vi "Check Test Report.vi"(8 "error in (no error)":errorcluster) -> (0 "error out":errorcluster)   [LabVIEW 2021]
uses:
  <vilib>/addons/_JKI Toolkits/Caraya/classes/Properties.Test/Properties.Test.lvclass
  C:/Program Files (x86)/National Instruments/LabVIEW 2021/vi.lib/addons/_JKI Toolkits/Caraya/classes/Properties/Properties.lvclass
  <vilib>/addons/_JKI Toolkits/Caraya/classes/Properties.Assert/Properties.Assert.lvclass
  <vilib>/Utility/file.llb/Read Delimited Spreadsheet (string).vi
  <vilib>/addons/_JKI Toolkits/Caraya/classes/Assert/Assert Equal Value_Variant.vi
  <vilib>/addons/_JKI Toolkits/Caraya/classes/Assert/Assert Greater Or Equal_Variant.vi
  <vilib>/addons/_JKI Toolkits/Caraya/classes/Assert/Assert True.vi
  <vilib>/addons/_JKI Toolkits/Caraya/classes/Test/Test.lvclass
  <vilib>/addons/_JKI Toolkits/Caraya/classes/Assert/Assert.lvclass
  <vilib>/addons/_JKI Toolkits/Caraya/classes/Properties/Properties.lvclass
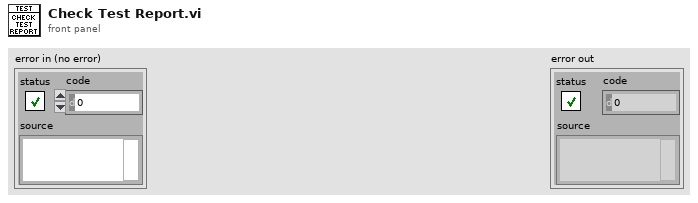
[diagram p1: front panel]
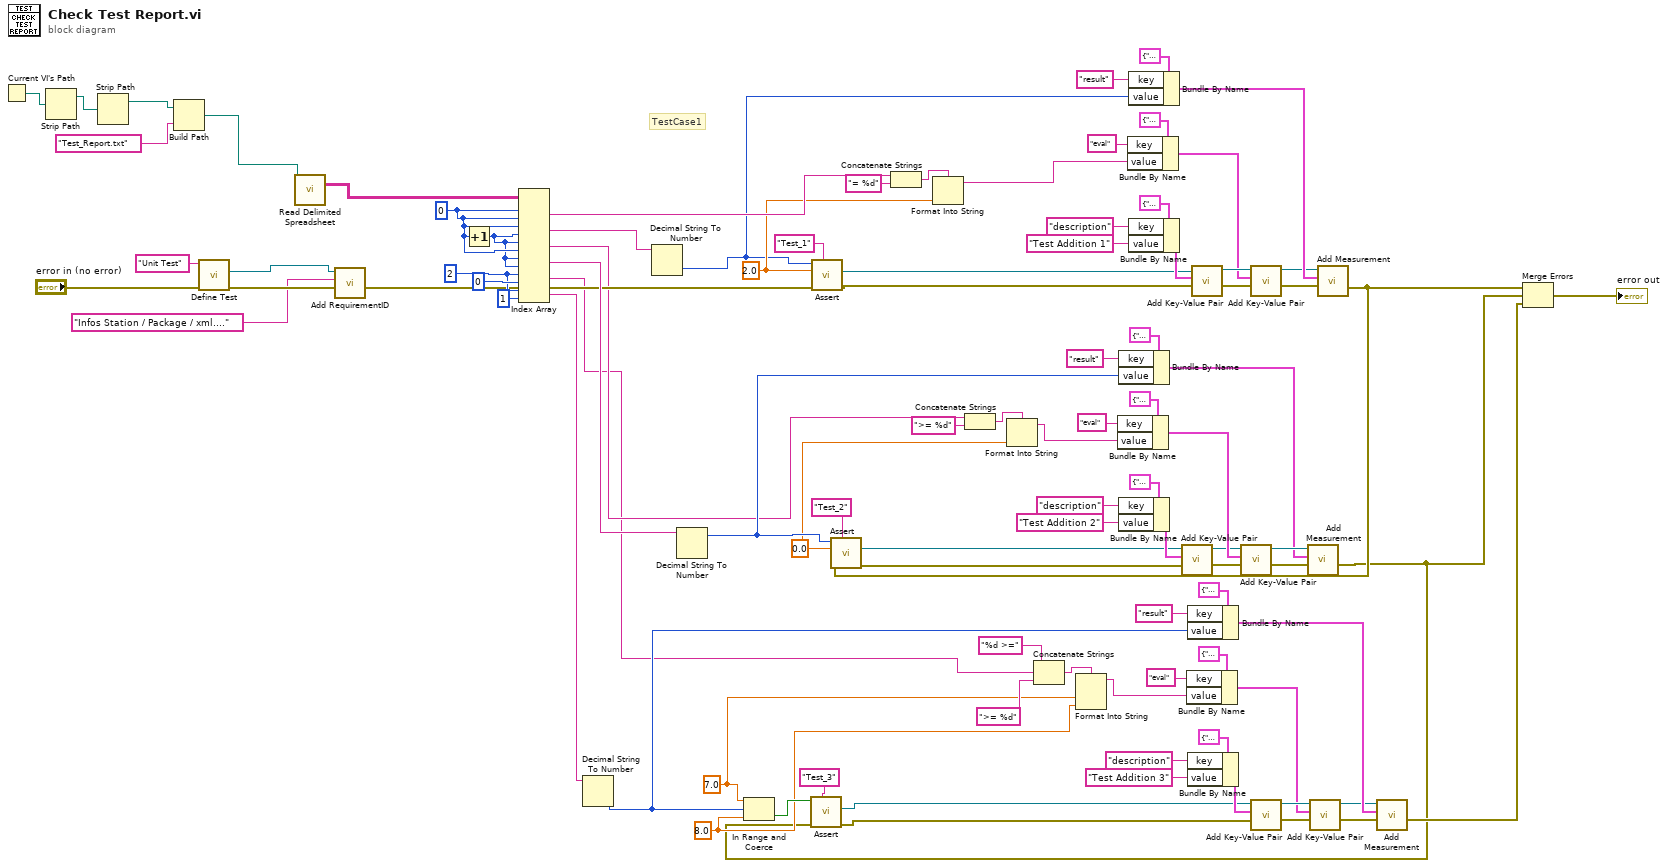
[diagram p0: block diagram]
diagram:
  w88 = 2 ("indice (ligne)")
  w92 = 0 ("indice (ligne)")
  w13 = 7.0 ("x+y")
  w12 = 8.0 ("x+y")
  w38 = 0.0 ("x+y")
  w63 = 2.0 ("x+y")
  # "TestCase1"
  n1 = Current VI's Path() -> (path=w5:path)
  n2 = Strip Path(path=w5) -> (stripped path=w4:path)  [unwired: 1 out]
  n3 = Strip Path(path=w4) -> (stripped path=w3:path)  [unwired: 1 out]
  n4 = Build Path(base path=w3, name or relative path="Test_Report.txt") -> (appended path=w1:path)
  n5 = call <vilib>:"Define Test.vi"("error in (no error)"="error in (no error)", "Label (VI Title)"="Unit Test") -> ("error out"=w84:errorcluster, "Properties.Test"=w58:refnum<class "Properties.Test.lvclass">)  [unwired: 8 in]
  n6 = call-poly <vilib>:"Read Delimited Spreadsheet.vi"("file path (dialog if empty)"=w1) -> ("all rows"=w93:string[][])  [unwired: 9 in, 5 out]
  n7 = call <vilib>:"Add RequirementID.vi"("error in (no error)"=w84, "Requirement ID"="Infos Station / Package / xml....", "Properties"=w58) -> ("error out"=w83:errorcluster)  [unwired: 7 in, 1 out]
  n8 = Increment(x=w92) -> (x+1=w91:i32)
  n9 = Index Array(array=w93, index (row) #1=w92, index (col) #1=w92, index (row) #2=w92, index (col) #2=w91, index (row) #3=w91, index (col) #3=w92, index (row) #4=w91, index (col) #4=w91, index (row) #5=w88, index (col) #5=0 ("indice désactivé (col)"), index (row) #6=w88, index (col) #6=1 ("indice désactivé (col)")) -> (element #1=w67:string, element #2=w65:string, element #3=w37:string, element #4=w90:string, element #5=w15:string, element #6=w86:string)
  n10 = Decimal String To Number(string=w86) -> (number=w16:i32)  [unwired: 2 in, 1 out]
  n11 = Decimal String To Number(string=w65) -> (number=w61:i32)  [unwired: 2 in, 1 out]
  n12 = Decimal String To Number(string=w90) -> (offset past number=w41:i32)  [unwired: 2 in, 1 out]
  n13 = In Range and Coerce(upper limit=w13, x=w16, lower limit=w12) -> (In Range?=w85:bool)  [unwired: 1 out]
  n14 = call-poly <vilib>:"Assert.vi"("Label"="Test_1", "error in (no error)"=w83, "Y"=w63, "X"=w61) -> ("error out"=w68:errorcluster, "Properties.Assert"=w60:refnum<class "Properties.Assert.lvclass">)  [unwired: 6 in]
  n15 = Concatenate Strings(w67, "= %d" ("chaîne")) -> (w8:string)
  n16 = Format Into String(format string=w8, w63) -> (resulting string=w62:string)  [unwired: 2 in, 1 out]
  n17 = Concatenate Strings(w37, ">= %d" ("chaîne")) -> (w9:string)
  n18 = Format Into String(format string=w9, w38) -> (resulting string=w39:string)  [unwired: 2 in, 1 out]
  n19 = Concatenate Strings("%d >=" ("chaîne"), w15, ">= %d" ("chaîne")) -> (w10:string)
  n20 = Format Into String(format string=w10, w13, w12) -> (resulting string=w35:string)  [unwired: 2 in, 1 out]
  n21 = Bundle By Name(cluster=cluster{"key":string, "value":variant} {"key"="", "value"=variant} ("entry"), "key"="eval", "value"=w39) -> (w56:cluster{"key":string, "value":variant})
  n22 = Bundle By Name(cluster=cluster{"key":string, "value":variant} {"key"="", "value"=variant} ("entry"), "key"="result", "value"=w41) -> (w50:cluster{"key":string, "value":variant})
  n23 = Bundle By Name(cluster=cluster{"key":string, "value":variant} {"key"="", "value"=variant} ("entry"), "key"="description", "value"="Test Addition 2" ("Label")) -> (w46:cluster{"key":string, "value":variant})
  n24 = Bundle By Name(cluster=cluster{"key":string, "value":variant} {"key"="", "value"=variant} ("entry"), "key"="eval", "value"=w62) -> (w70:cluster{"key":string, "value":variant})
  n25 = Bundle By Name(cluster=cluster{"key":string, "value":variant} {"key"="", "value"=variant} ("entry"), "key"="result", "value"=w61) -> (w76:cluster{"key":string, "value":variant})
  n26 = Bundle By Name(cluster=cluster{"key":string, "value":variant} {"key"="", "value"=variant} ("entry"), "key"="description", "value"="Test Addition 1" ("Label")) -> (w80:cluster{"key":string, "value":variant})
  n27 = Bundle By Name(cluster=cluster{"key":string, "value":variant} {"key"="", "value"=variant} ("entry"), "key"="eval", "value"=w35) -> (w21:cluster{"key":string, "value":variant})
  n28 = Bundle By Name(cluster=cluster{"key":string, "value":variant} {"key"="", "value"=variant} ("entry"), "key"="result", "value"=w16) -> (w27:cluster{"key":string, "value":variant})
  n29 = Bundle By Name(cluster=cluster{"key":string, "value":variant} {"key"="", "value"=variant} ("entry"), "key"="description", "value"="Test Addition 3" ("Label")) -> (w31:cluster{"key":string, "value":variant})
  n30 = call <vilib>:"Add Key-Value Pair.vi"("error in (no error)"=w68, "entry"=w80, "Properties in"=w60) -> ("error out"=w75:errorcluster, "Properties out"=w73:refnum<class "Properties.Assert.lvclass">)  [unwired: 7 in]
  n31 = call <vilib>:"Add Key-Value Pair.vi"("error in (no error)"=w75, "entry"=w70, "Properties in"=w73) -> ("error out"=w74:errorcluster, "Properties out"=w72:refnum<class "Properties.Assert.lvclass">)  [unwired: 7 in]
  n32 = call <vilib>:"Add Measurement.vi"("error in (no error)"=w74, "entry"=w76, "Properties"=w72) -> ("error out"=w7:errorcluster)  [unwired: 7 in, 1 out]
  n33 = call-poly <vilib>:"Assert.vi"("Label"="Test_2", "error in (no error)"=w7, "Y"=w38, "X"=w41) -> ("error out"=w43:errorcluster, "Properties.Assert"=w42:refnum<class "Properties.Assert.lvclass">)  [unwired: 6 in]
  n34 = call <vilib>:"Add Key-Value Pair.vi"("error in (no error)"=w43, "entry"=w46, "Properties in"=w42) -> ("error out"=w51:errorcluster, "Properties out"=w53:refnum<class "Properties.Assert.lvclass">)  [unwired: 7 in]
  n35 = call <vilib>:"Add Key-Value Pair.vi"("error in (no error)"=w51, "entry"=w56, "Properties in"=w53) -> ("error out"=w52:errorcluster, "Properties out"=w54:refnum<class "Properties.Assert.lvclass">)  [unwired: 7 in]
  n36 = call <vilib>:"Add Measurement.vi"("error in (no error)"=w52, "entry"=w50, "Properties"=w54) -> ("error out"=w6:errorcluster)  [unwired: 7 in, 1 out]
  n37 = call-poly <vilib>:"Assert.vi"("Label"="Test_3", "error in (no error)"=w6, "True?"=w85) -> ("error out"=w19:errorcluster, "Properties"=w18:refnum<class "Properties.Assert.lvclass">)  [unwired: 7 in]
  n38 = call <vilib>:"Add Key-Value Pair.vi"("error in (no error)"=w19, "entry"=w31, "Properties in"=w18) -> ("error out"=w26:errorcluster, "Properties out"=w24:refnum<class "Properties.Assert.lvclass">)  [unwired: 7 in]
  n39 = call <vilib>:"Add Key-Value Pair.vi"("error in (no error)"=w26, "entry"=w21, "Properties in"=w24) -> ("error out"=w25:errorcluster, "Properties out"=w23:refnum<class "Properties.Assert.lvclass">)  [unwired: 7 in]
  n40 = call <vilib>:"Add Measurement.vi"("error in (no error)"=w25, "entry"=w27, "Properties"=w23) -> ("error out"=w17:errorcluster)  [unwired: 7 in, 1 out]
  n41 = Merge Errors(w7, w6, w17) -> (→"error out":errorcluster)
